vi "generateWaveform.vi"(8 "error in (no error)":errorcluster, 11 "PeriodicWave in":refnum<class "PeriodicWave.lvclass">) -> (0 "error out":errorcluster, 2 "Signal Out":dbl, 3 "PeriodicWave out":refnum<class "PeriodicWave.lvclass">)   [LabVIEW 2015, in "PeriodicWave.lvclass"]
uses:
  PeriodicWave.lvclass
  PeriodicWave.lvclass/PeriodicWave.ctl
  <vilib>/measure/NI_MABase.lvlib
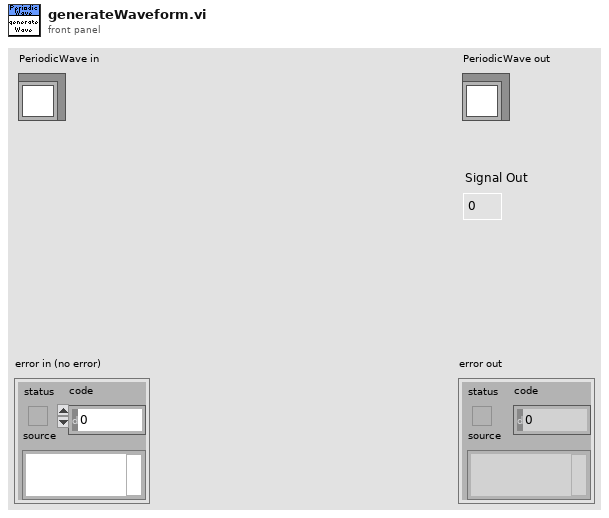
[diagram p1: front panel]
types:
  T1 = enum16{"Sine Wave", "Triangle Wave", "Square Wave", "Sawtooth Wave"}
  T2 = typedef "FAMTTypedefs.lvlib/DutyCycle.ctl" = dbl
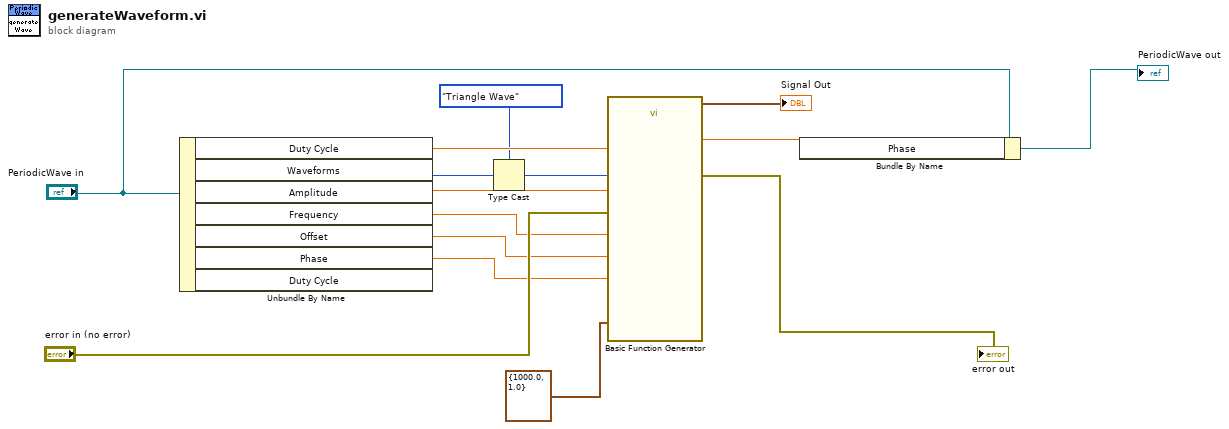
[diagram p0: block diagram]
diagram:
  n1 = Unbundle By Name("PeriodicWave in") -> ("Duty Cycle"=w4:T2, "Waveforms"=w2:u16, "Amplitude"=w12:dbl, "Frequency"=w11:dbl, "Offset"=w10:dbl, "Phase"=w9:dbl)  [unwired: 1 out]
  n2 = Type Cast(type=T1."Triangle Wave" ("signal type"), x=w2) -> (*(type *) &x=w1:T1)
  n3 = call <vilib>:"Basic Function Generator.vi"("offset"=w10, "square wave duty cycle (%)"=w4, "sampling info"=cluster{"Fs":dbl, "#s":dbl} {"Fs"=1000.0, "#s"=1.0}, "signal type"=w1, "error in (no error)"="error in (no error)", "phase"=w9, "amplitude"=w12, "frequency"=w11) -> ("error out"=→"error out":errorcluster, "phase out"=w7:dbl, "signal out"=→"Signal Out":waveform(dbl))  [unwired: 1 in]
  n4 = Bundle By Name(cluster="PeriodicWave in", "Phase"=w7) -> (→"PeriodicWave out":refnum<class "PeriodicWave.lvclass">)
